vi "Convert Humidity.vi"(8 "Chamber Temperature":dbl, 9 "Processed Variables 3":T1 {"Chamber Temperature" format="%.2f"; "Ambient Temperature" format="%.2f"; "Bath Temperature" format="%.2f"; "Det. Temperature" format="%.2f"; "Detector Chl 4" format="%.2g"; "Detector Chl 3" format="%.2g"; "Ref CO2" format="%.2g"; "Detector Chl 2" format="%.2g"; "Film Temperature" format="%.2f"; "Humidity" format="%.2f"; "Detector Chl 1" format="%.2g"}, 10 "Raw Voltage":dbl) -> (2 "Processed Variables 2":T1 {"Chamber Temperature" format="%.2f"; "Ambient Temperature" format="%.2f"; "Bath Temperature" format="%.2f"; "Det. Temperature" format="%.2f"; "Detector Chl 4" format="%.2g"; "Detector Chl 3" format="%.2g"; "Ref CO2" format="%.2g"; "Detector Chl 2" format="%.2g"; "Film Temperature" format="%.2f"; "Humidity" format="%.2f"; "Detector Chl 1" format="%.2g"}, 4 "Humidity":dbl)   [LabVIEW 2016]
uses:
  Controls/Processed Variables.ctl
  Miscellaneous/Globals.vi
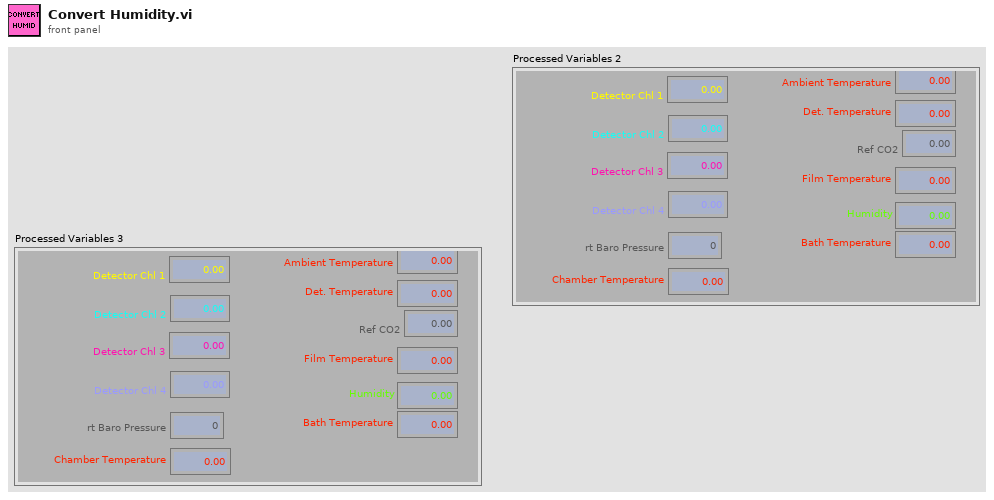
[diagram p1: front panel]
types:
  T1 = typedef "Processed Variables.ctl" = cluster{"Detector Chl 1":sgl, "Humidity":dbl, "Film Temperature":dbl, "Detector Chl 2":sgl, "Ref CO2":sgl, "Detector Chl 3":sgl, "Detector Chl 4":sgl, "Det. Temperature":dbl, "Bath Temperature":dbl, "Ambient Temperature":dbl, "rt Baro Pressure":u16, "Chamber Temperature":dbl}
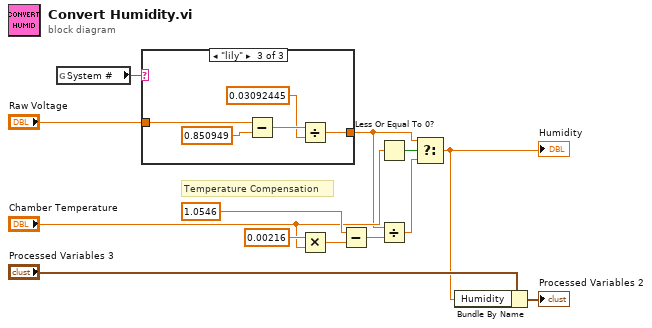
[diagram p0: block diagram]
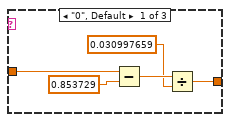
[diagram p2: hidden frame]
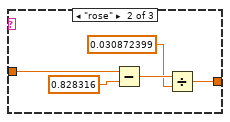
[diagram p3: hidden frame]
diagram:
  # "Temperature Compensation"
  n1 = global read "Globals.vi" "System #"() -> (w4:string)
  n2 = case shown="\"lily\"" w4 {
    tunnel: "Raw Voltage" -> [w17 w22 w27]
    tunnel: [w16 w21 w26] -> w6
    frame "0", Default {
      n3 = Subtract(x=w17, y=0.853729) -> (x-y=w18:dbl)
      n4 = Divide(x=w18, y=0.030997659) -> (x/y=w16:dbl)
    }
    frame "rose" {
      n5 = Subtract(x=w22, y=0.828316) -> (x-y=w23:dbl)
      n6 = Divide(x=w23, y=0.030872399) -> (x/y=w21:dbl)
    }
    frame "lily" {
      n7 = Subtract(x=w27, y=0.850949) -> (x-y=w28:dbl)
      n8 = Divide(x=w28, y=0.03092445) -> (x/y=w26:dbl)
    }
  }
  n9 = Multiply(x=0.00216 ("y"), y="Chamber Temperature") -> (x*y=w10:dbl)
  n10 = Subtract(x=1.0546 ("y"), y=w10) -> (x-y=w5:dbl)
  n11 = Less Or Equal To 0?(x="Chamber Temperature") -> (x <= 0?=w12:bool)
  n12 = Divide(x=w6, y=w5) -> (x/y=w7:dbl)
  n13 = Select(t=w6, s=w12, f=w7) -> (s? t:f=w1:dbl)
  "Humidity" <- w1
  n14 = Bundle By Name(cluster="Processed Variables 3", "Humidity"=w1) -> (→"Processed Variables 2":T1)
